vi "AUTON_Index.vi"(0 "Auton Array":dbl[][](array[numeric]), 5 "MeasuredHeading":dbl, 7 "LeftEncoder":dbl, 9 "RightEncoder":dbl) -> (4 "Right Drive":dbl, 6 "Left Drive":dbl, 8 "Harvester":dbl, 10 "Winch":dbl, 14 "Roller":dbl, 15 "Cam":dbl)   [LabVIEW 2013]
uses:
  Robot Global Data.vi
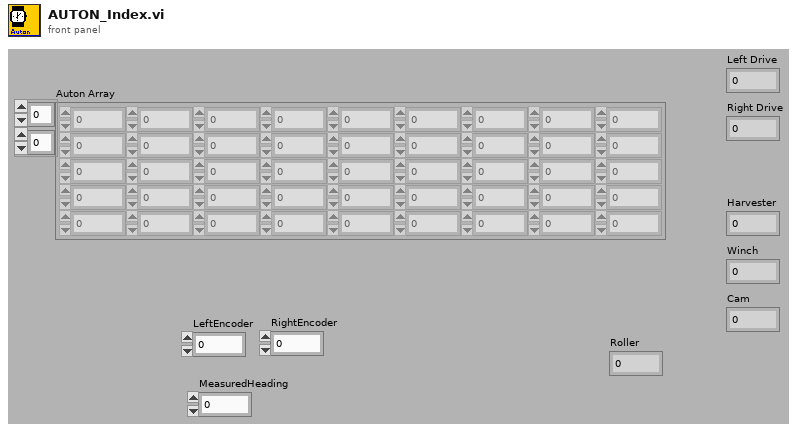
[diagram p1: front panel]
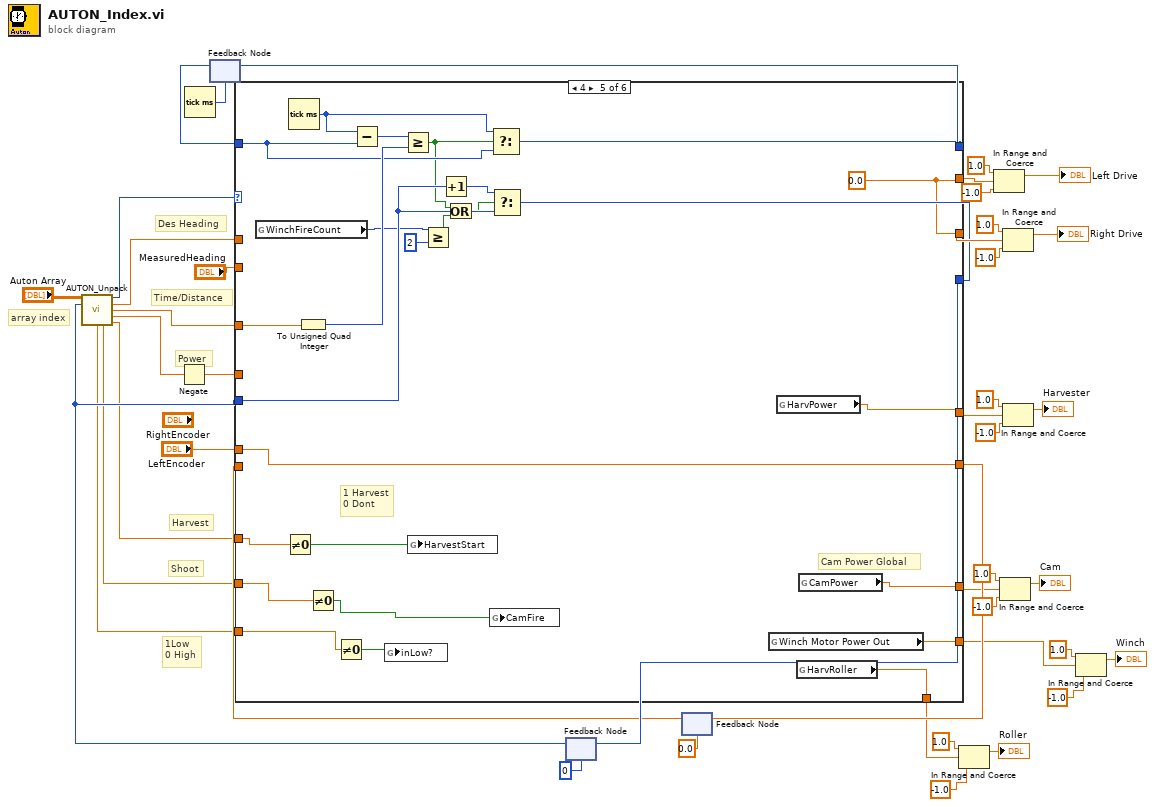
[diagram p0: block diagram]
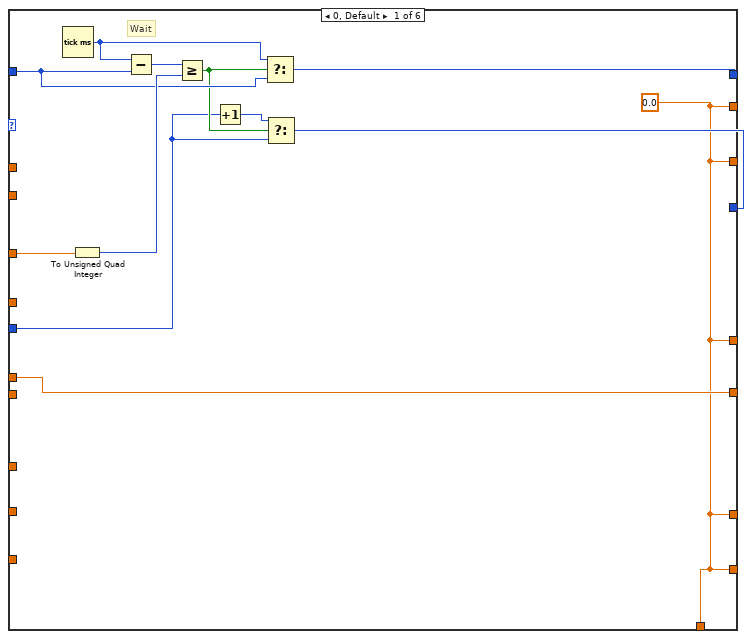
[diagram p2: hidden frame]
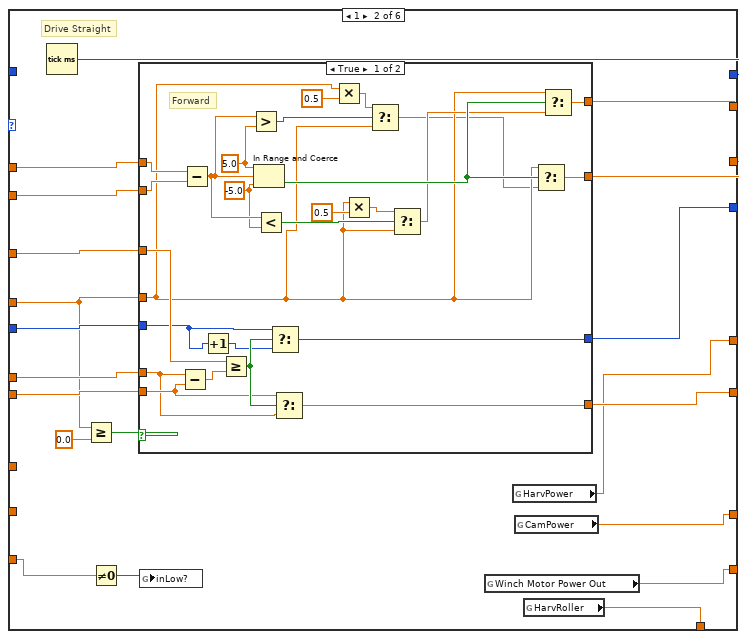
[diagram p3: hidden frame]
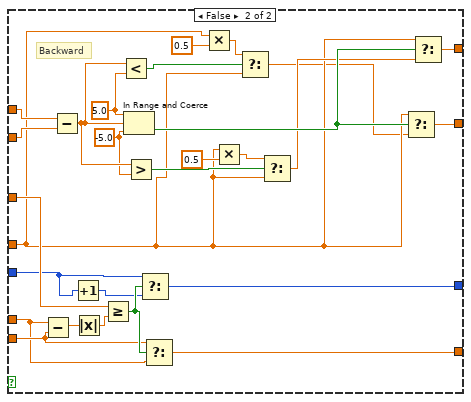
[diagram p4: hidden frame]
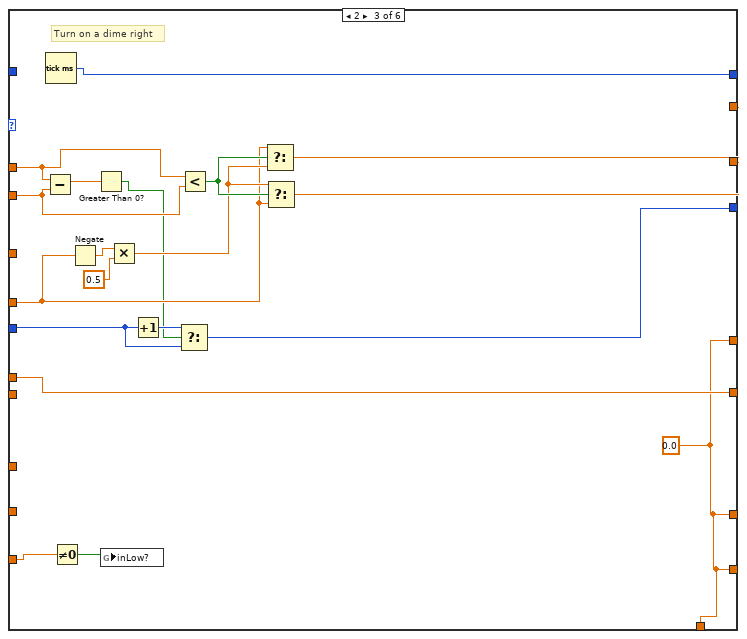
[diagram p5: hidden frame]
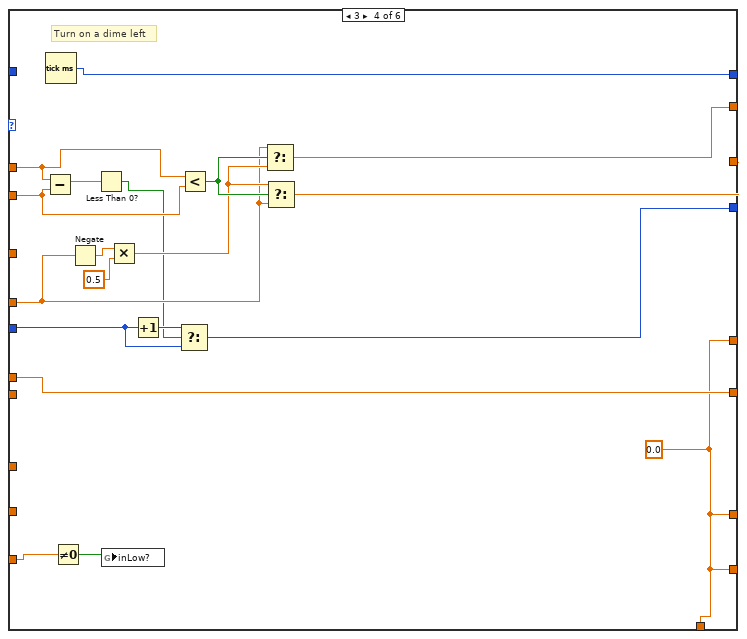
[diagram p6: hidden frame]
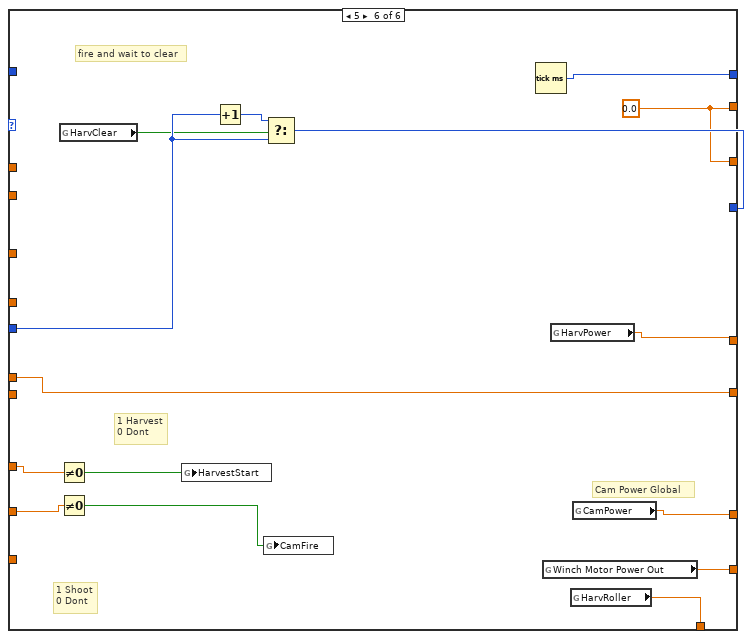
[diagram p7: hidden frame]
diagram:
  # "1Low\n0 High"
  # "Shoot"
  # "Harvest"
  # "Des Heading"
  # "Time/Distance"
  # "Power"
  # "array index"
  n1 = Tick Count (ms)() -> (millisecond timer value=w42:u32)
  n2 = feedback #1(w42) -> (w43:u32)
  n3 = feedback #2(0) -> (w23:i32)
  n4 = call "AUTON_Unpack.vi"("all rows"="Auton Array", "Index"=w23) -> ("Primitive ID"=w26:i16, "Desired Heading"=w25:dbl, "Time/Distance"=w24:dbl, "Power"=w11:dbl, "LowGear"=w1:dbl, "Shoot"=w8:dbl, "Harvest"=w9:dbl)  [unwired: 7 in]
  n5 = Negate(x=w11) -> (-x=w10:dbl)
  n6 = feedback #3(0.0) -> (w28:dbl)
  n7 = case shown="4" w26 {
    tunnel: [w48 w74 w143 w162 w186 w206] -> w30
    tunnel: w23 -> [w49 w69 w146 w165 w187 w207]
    tunnel: [w56 w66 w148 w167 w193 w197] -> w32
    tunnel: w43 -> [w53 _ _ _ w190 _]
    tunnel: w24 -> [w47 w75 _ _ w185 _]
    tunnel: w25 -> [_ w73 w141 w160 _ _]
    tunnel: [w45 w71 w144 w163 w184 w205] -> w40
    tunnel: [w45 w70 w145 w164 w184 w205] -> w33
    tunnel: w10 -> [_ w65 w135 w154 _ _]
    tunnel: "LeftEncoder" -> [w46 w67 w142 w161 w183 w204]
    tunnel: "MeasuredHeading" -> [_ w72 w140 w159 _ _]
    tunnel: w28 -> [_ w68 _ _ _ _]
    tunnel: [w46 w76 w142 w161 w183 w204] -> w27
    tunnel: [w45 w62 w132 w151 w181 w202] -> w13
    tunnel: [w45 w60 w132 w151 w182 w203] -> w12
    tunnel: w9 -> [_ _ _ _ w178 w200]
    tunnel: w8 -> [_ _ _ _ w180 w195]
    tunnel: [w45 w61 w132 w151 w179 w201] -> w7
    tunnel: [w45 w59 w132 w151 w175 w198] -> w3
    tunnel: w1 -> [_ w57 w130 w149 w168 _]
    frame 0, Default {
      w45 = 0.0 ("Numeric")
      # "Wait"
      n8 = Tick Count (ms)() -> (millisecond timer value=w52:u32)
      n9 = To Unsigned Quad Integer(1:w47) -> (0:w54:u64)
      n10 = Subtract(x=w52, y=w53) -> (x-y=w55:u32)
      n11 = Greater Or Equal?(x=w55, y=w54) -> (x >= y?=w51:bool)
      n12 = Increment(x=w49) -> (x+1=w50:i32)
      n13 = Select(t=w52, s=w51, f=w53) -> (s? t:f=w56:u32)
      n14 = Select(t=w50, s=w51, f=w49) -> (s? t:f=w48:i32)
    }
    frame 1 {
      # "Drive Straight"
      n15 = Tick Count (ms)() -> (millisecond timer value=w66:u32)
      n16 = Greater Or Equal?(x=w65, y=0.0) -> (x >= y?=w63:bool)
      n17 = Not Equal To 0?(x=w57) -> (x != 0?=w58:bool)
      n18 = case shown="True" w63 {
        tunnel: [w102 w129] -> w76
        tunnel: w75 -> [w100 w128]
        tunnel: [w98 w126] -> w74
        tunnel: w73 -> [w97 w125]
        tunnel: w72 -> [w96 w124]
        tunnel: [w94 w122] -> w71
        tunnel: [w93 w121] -> w70
        tunnel: w65 -> [w82 w110]
        tunnel: w69 -> [w79 w107]
        tunnel: w68 -> [w78 w106]
        tunnel: w67 -> [w77 w105]
        frame True {
          w90 = -5.0 ("lower limit")
          w92 = 5.0 ("upper limit")
          # "Forward"
          n19 = Subtract(x=w77, y=w78) -> (x-y=w101:dbl)
          n20 = Subtract(x=w97, y=w96) -> (x-y=w91:dbl)
          n21 = Increment(x=w79) -> (x+1=w80:i32)
          n22 = Greater Or Equal?(x=w100, y=w101) -> (x >= y?=w99:bool)
          n23 = Greater?(x=w91, y=w92) -> (0:w85:bool)
          n24 = In Range and Coerce(upper limit=w92, x=w91, lower limit=w90) -> (In Range?=w95:bool)  [unwired: 1 out]
          n25 = Less?(x=w91, y=w90) -> (x < y?=w89:bool)
          n26 = Select(t=w79, s=w99, f=w80) -> (s? t:f=w98:i32)
          n27 = Select(t=w78, s=w99, f=w77) -> (s? t:f=w102:dbl)
          n28 = Multiply(x=w82, y=0.5) -> (x*y=w84:dbl)
          n29 = Multiply(x=w82, y=0.5) -> (x*y=w87:dbl)
          n30 = Select(t=w84, s=w85, f=w82) -> (s? t:f=w81:dbl)
          n31 = Select(t=w87, s=w89, f=w82) -> (s? t:f=w86:dbl)
          n32 = Select(t=w82, s=w95, f=w81) -> (s? t:f=w93:dbl)
          n33 = Select(t=w82, s=w95, f=w86) -> (s? t:f=w94:dbl)
        }
        frame False {
          w118 = -5.0 ("lower limit")
          w120 = 5.0 ("upper limit")
          # "Backward"
          n34 = Subtract(x=w105, y=w106) -> (x-y=w103:dbl)
          n35 = Subtract(x=w125, y=w124) -> (x-y=w119:dbl)
          n36 = Increment(x=w107) -> (x+1=w108:i32)
          n37 = Absolute Value(x=w103) -> (abs(x)=w104:dbl)
          n38 = Greater Or Equal?(x=w128, y=w104) -> (x >= y?=w127:bool)
          n39 = Less?(x=w119, y=w120) -> (x < y?=w113:bool)
          n40 = In Range and Coerce(upper limit=w120, x=w119, lower limit=w118) -> (In Range?=w123:bool)  [unwired: 1 out]
          n41 = Greater?(x=w119, y=w118) -> (0:w117:bool)
          n42 = Select(t=w107, s=w127, f=w108) -> (s? t:f=w126:i32)
          n43 = Select(t=w106, s=w127, f=w105) -> (s? t:f=w129:dbl)
          n44 = Multiply(x=w110, y=0.5) -> (x*y=w112:dbl)
          n45 = Multiply(x=w110, y=0.5) -> (x*y=w115:dbl)
          n46 = Select(t=w112, s=w113, f=w110) -> (s? t:f=w109:dbl)
          n47 = Select(t=w115, s=w117, f=w110) -> (s? t:f=w114:dbl)
          n48 = Select(t=w110, s=w123, f=w109) -> (s? t:f=w121:dbl)
          n49 = Select(t=w110, s=w123, f=w114) -> (s? t:f=w122:dbl)
        }
      }
      n50 = global write "Robot Global Data.vi" "inLow?"(w58) -> ()
      n51 = global read "Robot Global Data.vi" "Winch Motor Power Out"() -> (w61:dbl)
      n52 = global read "Robot Global Data.vi" "HarvPower"() -> (w60:dbl)
      n53 = global read "Robot Global Data.vi" "CamPower"() -> (w62:dbl)
      n54 = global read "Robot Global Data.vi" "HarvRoller"() -> (w59:dbl)
    }
    frame 2 {
      w132 = 0.0 ("Numeric")
      # "Turn on a dime right"
      n55 = Subtract(x=w141, y=w140) -> (x-y=w134:dbl)
      n56 = Tick Count (ms)() -> (millisecond timer value=w148:u32)
      n57 = Not Equal To 0?(x=w130) -> (x != 0?=w131:bool)
      n58 = Negate(x=w135) -> (-x=w138:dbl)
      n59 = Greater Than 0?(x=w134) -> (x > 0?=w133:bool)
      n60 = global write "Robot Global Data.vi" "inLow?"(w131) -> ()
      n61 = Multiply(x=w138, y=0.5) -> (x*y=w136:dbl)
      n62 = Increment(x=w146) -> (x+1=w147:i32)
      n63 = Select(t=w147, s=w133, f=w146) -> (s? t:f=w143:i32)
      n64 = Less?(x=w141, y=w140) -> (x < y?=w139:bool)
      n65 = Select(t=w135, s=w139, f=w136) -> (s? t:f=w144:dbl)
      n66 = Select(t=w136, s=w139, f=w135) -> (s? t:f=w145:dbl)
    }
    frame 3 {
      w151 = 0.0 ("Numeric")
      # "Turn on a dime left"
      n67 = Subtract(x=w160, y=w159) -> (x-y=w153:dbl)
      n68 = Tick Count (ms)() -> (millisecond timer value=w167:u32)
      n69 = Not Equal To 0?(x=w149) -> (x != 0?=w150:bool)
      n70 = Negate(x=w154) -> (-x=w157:dbl)
      n71 = Less Than 0?(x=w153) -> (x < 0?=w152:bool)
      n72 = global write "Robot Global Data.vi" "inLow?"(w150) -> ()
      n73 = Multiply(x=w157, y=0.5) -> (x*y=w155:dbl)
      n74 = Increment(x=w165) -> (x+1=w166:i32)
      n75 = Select(t=w166, s=w152, f=w165) -> (s? t:f=w162:i32)
      n76 = Less?(x=w160, y=w159) -> (x < y?=w158:bool)
      n77 = Select(t=w154, s=w158, f=w155) -> (s? t:f=w163:dbl)
      n78 = Select(t=w155, s=w158, f=w154) -> (s? t:f=w164:dbl)
    }
    frame 4 {
      w184 = 0.0 ("Numeric")
      # "1 Harvest\n0 Dont"
      # "Cam Power Global"
      n79 = global read "Robot Global Data.vi" "WinchFireCount"() -> (w171:i32)
      n80 = Not Equal To 0?(x=w178) -> (x != 0?=w177:bool)
      n81 = Tick Count (ms)() -> (millisecond timer value=w189:u32)
      n82 = To Unsigned Quad Integer(1:w185) -> (0:w191:u64)
      n83 = Not Equal To 0?(x=w180) -> (x != 0?=w176:bool)
      n84 = Not Equal To 0?(x=w168) -> (x != 0?=w169:bool)
      n85 = Subtract(x=w189, y=w190) -> (x-y=w192:u32)
      n86 = global write "Robot Global Data.vi" "inLow?"(w169) -> ()
      n87 = Greater Or Equal?(x=w192, y=w191) -> (x >= y?=w173:bool)
      n88 = global write "Robot Global Data.vi" "HarvestStart"(w177) -> ()
      n89 = Greater Or Equal?(x=w171, y=2) -> (x >= y?=w172:bool)
      n90 = Increment(x=w187) -> (x+1=w188:i32)
      n91 = Or(x=w173, y=w172) -> (x .or. y?=w174:bool)
      n92 = global write "Robot Global Data.vi" "CamFire"(w176) -> ()
      n93 = Select(t=w189, s=w173, f=w190) -> (s? t:f=w193:u32)
      n94 = Select(t=w188, s=w174, f=w187) -> (s? t:f=w186:i32)
      n95 = global read "Robot Global Data.vi" "Winch Motor Power Out"() -> (w179:dbl)
      n96 = global read "Robot Global Data.vi" "HarvPower"() -> (w182:dbl)
      n97 = global read "Robot Global Data.vi" "HarvRoller"() -> (w175:dbl)
      n98 = global read "Robot Global Data.vi" "CamPower"() -> (w181:dbl)
    }
    frame 5 {
      w205 = 0.0 ("Numeric")
      # "fire and wait to clear"
      # "1 Harvest\n0 Dont"
      # "1 Shoot\n0 Dont"
      # "Cam Power Global"
      n99 = Not Equal To 0?(x=w200) -> (x != 0?=w199:bool)
      n100 = Not Equal To 0?(x=w195) -> (x != 0?=w194:bool)
      n101 = global read "Robot Global Data.vi" "HarvClear"() -> (w196:bool)
      n102 = global write "Robot Global Data.vi" "HarvestStart"(w199) -> ()
      n103 = Increment(x=w207) -> (x+1=w208:i32)
      n104 = global write "Robot Global Data.vi" "CamFire"(w194) -> ()
      n105 = Select(t=w208, s=w196, f=w207) -> (s? t:f=w206:i32)
      n106 = Tick Count (ms)() -> (millisecond timer value=w197:u32)
      n107 = global read "Robot Global Data.vi" "Winch Motor Power Out"() -> (w201:dbl)
      n108 = global read "Robot Global Data.vi" "HarvPower"() -> (w203:dbl)
      n109 = global read "Robot Global Data.vi" "HarvRoller"() -> (w198:dbl)
      n110 = global read "Robot Global Data.vi" "CamPower"() -> (w202:dbl)
    }
  }
  n111 = feedback-in #1(w32) -> ()
  n112 = feedback-in #2(w30) -> ()
  n113 = feedback-in #3(w27) -> ()
  n114 = In Range and Coerce(upper limit=1.0, x=w3, lower limit=-1.0) -> (coerced(x)=→"Roller":dbl)  [unwired: 1 out]
  n115 = In Range and Coerce(upper limit=1.0, x=w40, lower limit=-1.0) -> (coerced(x)=→"Left Drive":dbl)  [unwired: 1 out]
  n116 = In Range and Coerce(upper limit=1.0, x=w13, lower limit=-1.0) -> (coerced(x)=→"Cam":dbl)  [unwired: 1 out]
  n117 = In Range and Coerce(upper limit=1.0, x=w33, lower limit=-1.0) -> (coerced(x)=→"Right Drive":dbl)  [unwired: 1 out]
  n118 = In Range and Coerce(upper limit=1.0, x=w12, lower limit=-1.0) -> (coerced(x)=→"Harvester":dbl)  [unwired: 1 out]
  n119 = In Range and Coerce(upper limit=1.0, x=w7, lower limit=-1.0) -> (coerced(x)=→"Winch":dbl)  [unwired: 1 out]
